vi "Create System Image (File).vi"(4 "File and Directory Blacklist":string[](array[string]), 5 "Encryption Passphrase":string, 6 "Overwrite (F)":bool, 7 "Restart Automatically (T)":bool=TRUE, 8 "error in (no error)":errorcluster, 9 "Image Metadata in":T1={"title"="", "description"="", "ID"="", "version"="", "component type"=5} {"component type" items=["standard", "hidden", "system", "unknown", "startup", "image", "essential"]}, 10 "Destination File":path, 11 "Session in":refnum<k21>) -> (0 "error out":errorcluster, 1 "Image Metadata out":T1={"title"="", "description"="", "ID"="", "version"="", "component type"=5} {"component type" items=["standard", "hidden", "system", "unknown", "startup", "image", "essential"]}, 3 "Session out":refnum<k21>)   [LabVIEW 2017, in "nisyscfg.lvlib"]
doc: "Creates a system image file—a copy of the file contents on a primary hard drive of a system in zip format. You may want to create a system image to restore a system to its original state or to deploy the image to other systems."
uses:
  <vilib>/nisyscfg/nisyscfg.lvlib
  <vilib>/nisyscfg/Software 1.2.ctl
  <vilib>/nisyscfg/Component Type.ctl
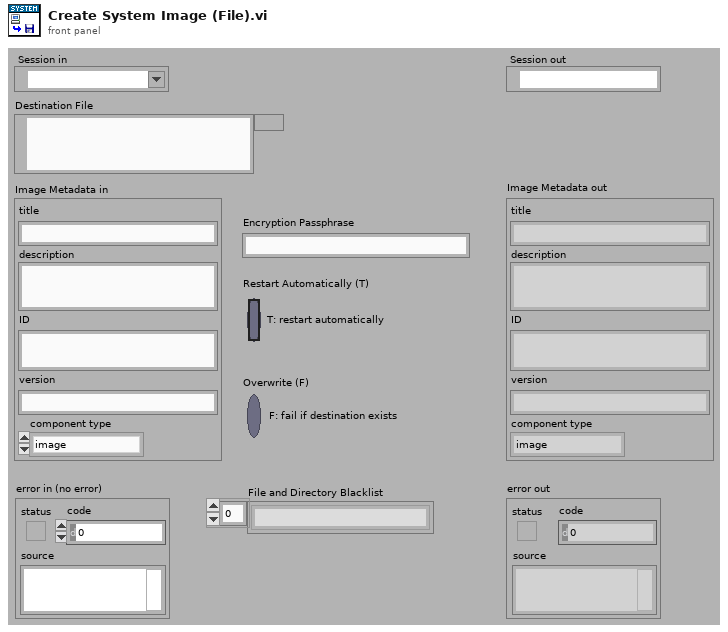
[diagram p1: front panel]
types:
  T1 = typedef "nisyscfg.lvlib/Software 1.2.ctl" = cluster{"title":string, "description":string, "ID":string, "version":string, "component type":T2}
  T2 = typedef "nisyscfg.lvlib/Component Type.ctl" = u32
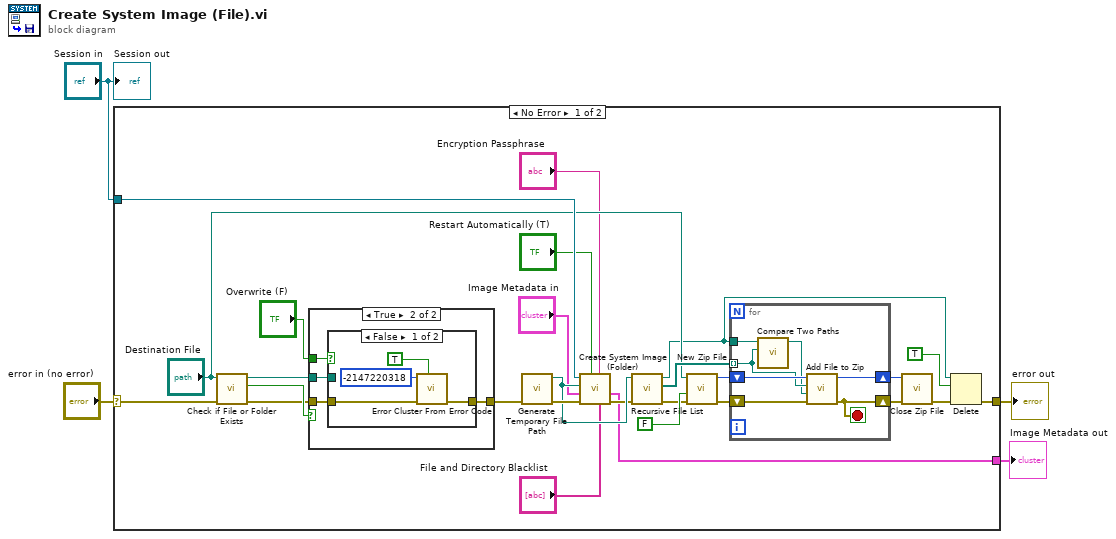
[diagram p0: block diagram]
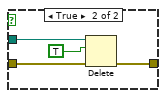
[diagram p3: hidden frame]
diagram:
  n1 = case shown="No Error" "error in (no error)" {
    selector: "error in (no error)" -> [w10 w52]
    tunnel: [w11 w52] -> w4
    tunnel: "Session in" -> [w25 _]
    tunnel: [w5 _] -> w1
    frame No Error {
      n2 = call <vilib>:"Check if File or Folder Exists.vi"("error in (no error)"=w10, "path"="Destination File") -> ("error out"=w28:errorcluster, "file or folder exists?"=w31:bool, "dup path"=w29:path)  [unwired: 7 in]
      n3 = case shown="True" w31 {
        tunnel: "Overwrite (F)" -> [_ w43]
        tunnel: w29 -> [_ w42]
        tunnel: [w39 w41] -> w27
        tunnel: w28 -> [w39 w40]
        frame False {
        }
        frame True {
          n4 = case shown="False" w43 {
            tunnel: w42 -> [_ w51]
            tunnel: [w46 w49] -> w41
            tunnel: w40 -> [w47 w48]
            frame False {
              n5 = call <vilib>:"Error Cluster From Error Code.vi"("show call chain? (False)"=TRUE, "error in (no error)"=w47, "error code (0)"=-2147220318) -> ("error out"=w46:errorcluster)  [unwired: 6 in]
            }
            frame True {
              n6 = Delete(path (use dialog)=w51, entire hierarchy (F)=TRUE, error in=w48) -> (error out=w49:errorcluster)  [unwired: 2 in, 2 out]
            }
          }
        }
      }
      n7 = call <vilib>:"Generate Temporary File Path.vi"("error in (no error)"=w27) -> ("error out"=w26:errorcluster, "Unique Temporary File Path"=w16:path)  [unwired: 9 in]
      n8 = call <vilib>:"Create System Image (Folder).vi"("File and Directory Blacklist"="File and Directory Blacklist", "Encryption Passphrase"="Encryption Passphrase", "Restart Automatically (T)"="Restart Automatically (T)", "error in (no error)"=w26, "Image Metadata in"="Image Metadata in", "Destination Folder"=w16, "Session in"=w25) -> ("error out"=w15:errorcluster, "Image Metadata out"=w5:T1)  [unwired: 2 in, 1 out]
      n9 = call <vilib>:"Recursive File List.vi"("error in (no error)"=w15, "Folder Path"=w16) -> ("error out"=w20:errorcluster, "All Files in Dir"=w22:path[], "dup Folder Path"=w12:path)  [unwired: 1 in, 6 out]
      n10 = call <vilib>:"New Zip File.vi"("error in (no error)"=w20, "confirm overwrite? (F)"=FALSE, "target"="Destination File") -> ("error out"=w23:errorcluster, "zip file out"=w24:i64)  [unwired: 3 out]
      n11 = for {
        tunnel: w22 -> [w34] mode=indexing
        shift-right: [w36] -> w18
        shift-left: w24 -> [w38]
        shift-right: [w35] -> w19
        shift-left: w23 -> [w37]
        tunnel: w12 -> [w32]
        stop <- w35 stop-if-true
        n12 = call <vilib>:"Compare Two Paths.vi"("Path 2"=w34, "Path 1"=w32) -> ("Relative Path from 1 to 2"=w33:path)  [unwired: 1 in, 8 out]
        n13 = call <vilib>:"Add File to Zip.vi"("error in (no error)"=w37, "destination path in zip"=w33, "source file path"=w34, "zip file in"=w38) -> ("error out"=w35:errorcluster, "zip file out"=w36:i64)  [unwired: 6 out]
      }
      n14 = call <vilib>:"Close Zip File.vi"("error in (no error)"=w19, "zip file in"=w18) -> ("error out"=w14:errorcluster)  [unwired: 1 in, 4 out]
      n15 = Delete(path (use dialog)=w12, entire hierarchy (F)=TRUE, error in=w14) -> (error out=w11:errorcluster)  [unwired: 2 in, 2 out]
    }
    frame Error {
    }
  }
  "error out" <- w4
  "Image Metadata out" <- w1
  "Session out" <- "Session in"
